vi "Delete TargetPanel by NodeRef.vi"(8 "error in":errorcluster caption="错误输入（无错误）", 9 "Abort VI":bool=TRUE, 10 "Node*":refnum<data-value>, 11 "PanelRootNode 输入":refnum<class "PanelRootNode.lvclass"> caption="DNL_LabVIEW Object in") -> (0 "error out":errorcluster caption="错误输出", 3 "PanelRootNode 输出":refnum<class "PanelRootNode.lvclass"> caption="DNL_LabVIEW Object out")   [LabVIEW 2016, in "PanelRootNode.lvclass"]
uses:
  PanelRootNode.lvclass
  C:/Users/CL/Desktop/ZcDAQprj0811/ZcDAQprj/Modules/DAQ-Display/PanelSplitToolkit/PanelLinkNode/PanelLinkNode.lvclass
  PanelObject/PanelObject.lvclass
  PanelLinkNode/PanelLinkNode.lvclass/PanelLinkNode.ctl
  PanelDataNode/PanelDataNode.lvclass
  C:/Users/CL/Desktop/ZcDAQprj0811/ZcDAQprj/Modules/DAQ-Display/PanelSplitToolkit/PanelObject/PanelObject.lvclass
  PanelLinkNode/PanelLinkNode.lvclass
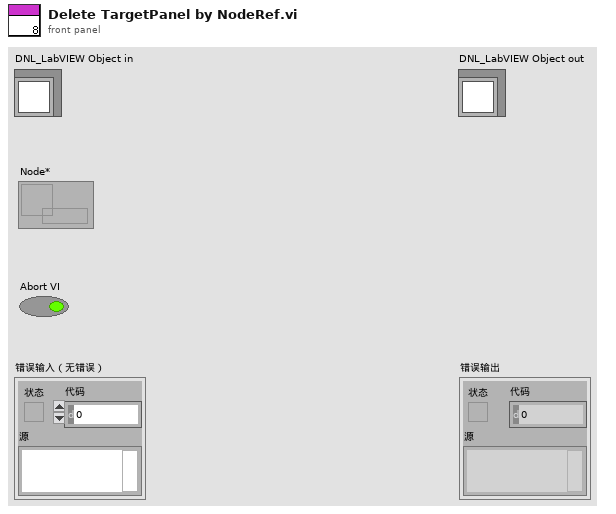
[diagram p1: front panel]
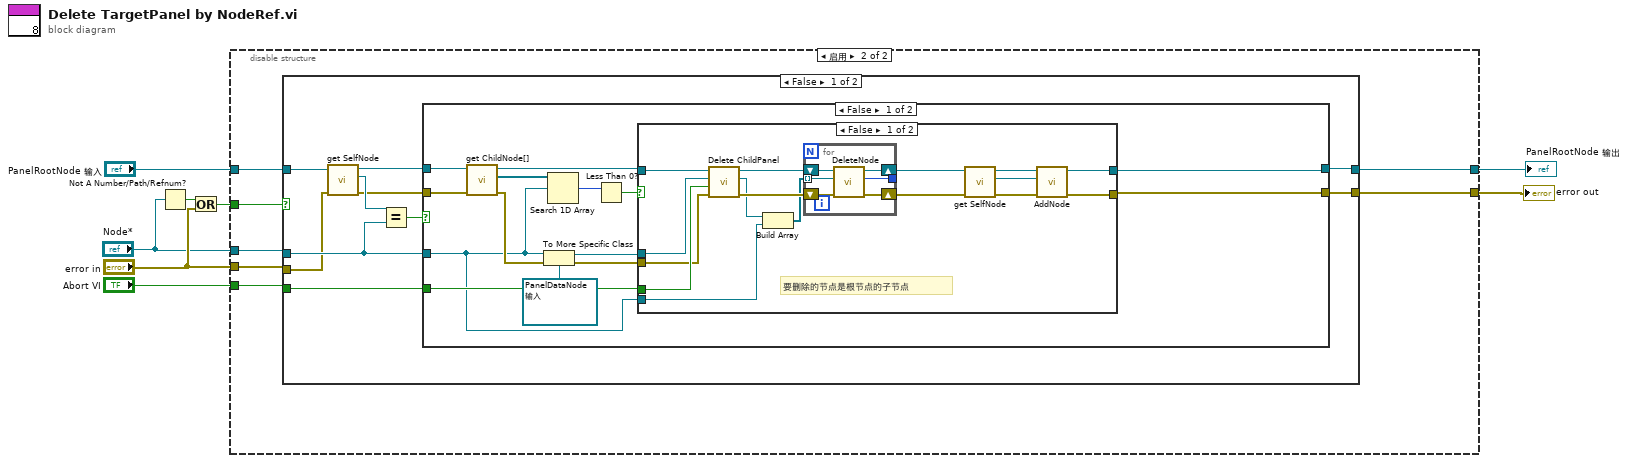
[diagram p0: block diagram]
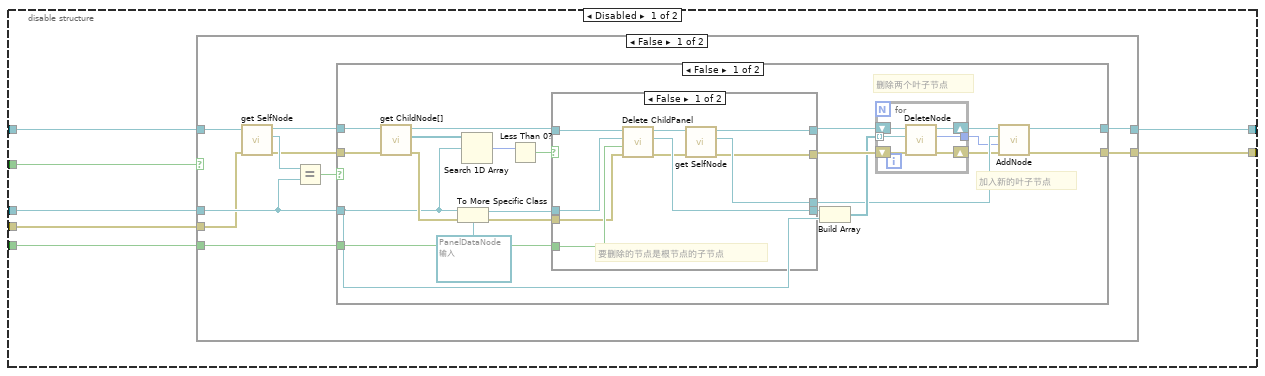
[diagram p2: hidden frame]
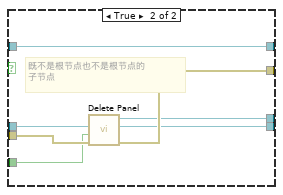
[diagram p3: hidden frame]
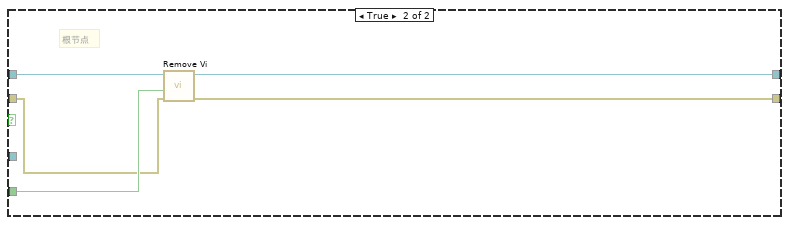
[diagram p4: hidden frame]
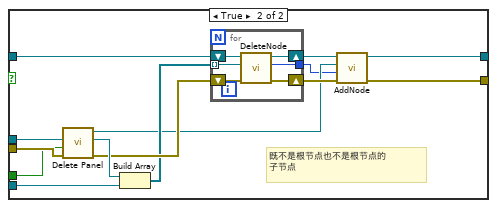
[diagram p6: hidden frame]
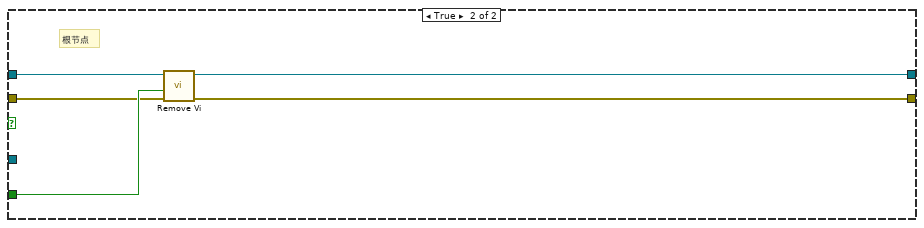
[diagram p7: hidden frame]
diagram:
  n1 = Not A Number/Path/Refnum?(number/path/refnum="Node*") -> (NaN/Path/Refnum?=w5:bool)
  n2 = Or(x=w5, y="error in") -> (x .or. y?=w4:bool)
  n3 = disable-structure shown="启用" {
    disable-tunnel: [w15 w82] -> w8
    disable-tunnel: "PanelRootNode 输入" -> [w14 w84]
    disable-tunnel: [w13 w83] -> w6
    disable-tunnel: w4 -> [w12 w78]
    disable-tunnel: "error in" -> [w11 w81]
    disable-tunnel: "Abort VI" -> [w10 w79]
    disable-tunnel: "Node*" -> [w9 w80]
    frame Disabled {
      n4 = case shown="False" w12 {
        tunnel: [w17 w76] -> w15
        tunnel: [w21 w77] -> w13
        tunnel: w14 -> [w25 w77]
        tunnel: w9 -> [w18 _]
        tunnel: w11 -> [w16 w76]
        tunnel: w10 -> [w20 _]
        frame False {
          n5 = call "get SelfNode.vi"("error in (no error)"=w16, "PanelLinkNode输入"=w25) -> ("error out"=w19:errorcluster, "SelfNode*"=w24:refnum<data-value>, "PanelLinkNode输出"=w23:refnum<class "PanelRootNode.lvclass">)  [unwired: 7 in]
          n6 = Equal?(x=w24, y=w18) -> (x = y?=w22:bool)
          n7 = case shown="False" w22 {
            tunnel: w23 -> [w47 w75]
            tunnel: [w30 w74] -> w21
            tunnel: w20 -> [w41 w73]
            tunnel: w19 -> [w46 w71]
            tunnel: w18 -> [w34 _]
            tunnel: [w26 w72] -> w17
            frame False {
              # "加入新的叶子节点"
              # "删除两个叶子节点"
              n8 = call "get ChildNode[].vi"("error in (no error)"=w46, "PanelLinkNode输入"=w47) -> ("error out"=w38:errorcluster, "ChildNode*[]"=w45:refnum<data-value>[], "PanelLinkNode输出"=w43:refnum<class "PanelRootNode.lvclass">)  [unwired: 7 in]
              n9 = To More Specific Class(target class=refnum<data-value> refnum ("数据值引用"), reference=w34, error in=w38) -> (specific class reference=w39:refnum<data-value>, error out=w37:errorcluster)
              n10 = Search 1D Array(1D array=w45, element=w34) -> (index of element=w44:i32)  [unwired: 1 in]
              n11 = Less Than 0?(x=w44) -> (x < 0?=w42:bool)
              n12 = case shown="False" w42 {
                tunnel: w43 -> [w63 w70]
                tunnel: [w57 w70] -> w36
                tunnel: w39 -> [w62 w69]
                tunnel: w41 -> [w61 w66]
                tunnel: w37 -> [w60 w68]
                tunnel: [w54 w67] -> w33
                tunnel: [w59 w65] -> w35
                tunnel: [w56 w64] -> w29
                frame False {
                  # "要删除的节点是根节点的子节点"
                  n13 = call-dynamic "Delete ChildPanel.vi"("error in"=w60, "Abort VI"=w61, "ChildNode*"=w62, "ParentNode in"=w63) -> ("error out"=w55:errorcluster, "AnotherChildNode*"=w59:refnum<data-value>, "Parent out"=w58:refnum<class "PanelRootNode.lvclass">)  [unwired: 5 in]
                  n14 = call "get SelfNode.vi"("error in (no error)"=w55, "PanelLinkNode输入"=w58) -> ("error out"=w54:errorcluster, "SelfNode*"=w56:refnum<data-value>, "PanelLinkNode输出"=w57:refnum<class "PanelRootNode.lvclass">)  [unwired: 7 in]
                }
                frame True {
                  # "既不是根节点也不是根节点的\n子节点"
                  n15 = call "Delete Panel.vi"("error in"=w68, "Abort VI"=w66, "SelfNode*"=w69) -> ("error out"=w67:errorcluster, "BrotherNodeBeDeleted"=w65:refnum<data-value>, "ParentNode*"=w64:refnum<data-value>)  [unwired: 6 in]
                }
              }
              n16 = Build Array(w35, w34) -> (w32:refnum<data-value>[])
              n17 = for {
                tunnel: w32 -> [w50] mode=indexing
                shift-right: [w52] -> w31
                shift-left: w36 -> [w53]
                shift-right: [w49] -> w27
                shift-left: w33 -> [w51]
                tunnel: [w48] -> w28
                n18 = call "DeleteNode.vi"("error in (no error)"=w51, "Node*"=w50, "PanelRootNode 输入"=w53) -> ("error out"=w49:errorcluster, "index"=w48:i32, "PanelRootNode 输出"=w52:refnum<class "PanelRootNode.lvclass">)  [unwired: 6 in]
              }
              n19 = call "AddNode.vi"("error in (no error)"=w27, "Index"=w28, "Node*"=w29, "PanelRootNode 输入"=w31) -> ("error out"=w26:errorcluster, "PanelRootNode 输出"=w30:refnum<class "PanelRootNode.lvclass">)  [unwired: 6 in]
            }
            frame True {
              # "根节点"
              n20 = call-dynamic "Remove Vi.vi"("error in"=w71, "Abort VI"=w73, "PanelDataNode 输入"=w75) -> ("error out"=w72:errorcluster, "PanelDataNode 输出"=w74:refnum<class "PanelRootNode.lvclass">)  [unwired: 5 in, 2 out]
            }
          }
        }
        frame True {
        }
      }
    }
    frame Enabled {
      n21 = case shown="False" w78 {
        tunnel: [w86 w156] -> w82
        tunnel: [w90 w157] -> w83
        tunnel: w84 -> [w94 w157]
        tunnel: w80 -> [w87 _]
        tunnel: w81 -> [w85 w156]
        tunnel: w79 -> [w89 _]
        frame False {
          n22 = call "get SelfNode.vi"("error in (no error)"=w85, "PanelLinkNode输入"=w94) -> ("error out"=w88:errorcluster, "SelfNode*"=w93:refnum<data-value>, "PanelLinkNode输出"=w92:refnum<class "PanelRootNode.lvclass">)  [unwired: 7 in]
          n23 = Equal?(x=w93, y=w87) -> (x = y?=w91:bool)
          n24 = case shown="False" w91 {
            tunnel: w92 -> [w108 w155]
            tunnel: [w96 w154] -> w90
            tunnel: w89 -> [w102 w153]
            tunnel: w88 -> [w107 w151]
            tunnel: w87 -> [w97 _]
            tunnel: [w95 w152] -> w86
            frame False {
              n25 = call "get ChildNode[].vi"("error in (no error)"=w107, "PanelLinkNode输入"=w108) -> ("error out"=w99:errorcluster, "ChildNode*[]"=w106:refnum<data-value>[], "PanelLinkNode输出"=w104:refnum<class "PanelRootNode.lvclass">)  [unwired: 7 in]
              n26 = To More Specific Class(target class=refnum<data-value> refnum ("数据值引用"), reference=w97, error in=w99) -> (specific class reference=w100:refnum<data-value>, error out=w98:errorcluster)
              n27 = Search 1D Array(1D array=w106, element=w97) -> (index of element=w105:i32)  [unwired: 1 in]
              n28 = Less Than 0?(x=w105) -> (x < 0?=w103:bool)
              n29 = case shown="False" w103 {
                tunnel: w104 -> [w124 w141]
                tunnel: [w109 w133] -> w96
                tunnel: w100 -> [w123 w144]
                tunnel: w102 -> [w122 w142]
                tunnel: w98 -> [w121 w143]
                tunnel: [w110 w134] -> w95
                tunnel: w97 -> [w117 w140]
                frame False {
                  # "要删除的节点是根节点的子节点"
                  n30 = call-dynamic "Delete ChildPanel.vi"("error in"=w121, "Abort VI"=w122, "ChildNode*"=w123, "ParentNode in"=w124) -> ("error out"=w119:errorcluster, "AnotherChildNode*"=w118:refnum<data-value>, "Parent out"=w120:refnum<class "PanelRootNode.lvclass">)  [unwired: 5 in]
                  n31 = Build Array(w118, w117) -> (w116:refnum<data-value>[])
                  n32 = for {
                    tunnel: w116 -> [w127] mode=indexing
                    shift-right: [w129] -> w115
                    shift-left: w120 -> [w130]
                    shift-right: [w126] -> w114
                    shift-left: w119 -> [w128]
                    tunnel: [w125] -> _
                    n33 = call "DeleteNode.vi"("error in (no error)"=w128, "Node*"=w127, "PanelRootNode 输入"=w130) -> ("error out"=w126:errorcluster, "index"=w125:i32, "PanelRootNode 输出"=w129:refnum<class "PanelRootNode.lvclass">)  [unwired: 6 in]
                  }
                  n34 = call "get SelfNode.vi"("error in (no error)"=w114, "PanelLinkNode输入"=w115) -> ("error out"=w111:errorcluster, "SelfNode*"=w112:refnum<data-value>, "PanelLinkNode输出"=w113:refnum<class "PanelRootNode.lvclass">)  [unwired: 7 in]
                  n35 = call "AddNode.vi"("error in (no error)"=w111, "Node*"=w112, "PanelRootNode 输入"=w113) -> ("error out"=w110:errorcluster, "PanelRootNode 输出"=w109:refnum<class "PanelRootNode.lvclass">)  [unwired: 7 in]
                }
                frame True {
                  # "既不是根节点也不是根节点的\n子节点"
                  n36 = call "Delete Panel.vi"("error in"=w143, "Abort VI"=w142, "SelfNode*"=w144) -> ("error out"=w138:errorcluster, "BrotherNodeBeDeleted"=w139:refnum<data-value>, "ParentNode*"=w132:refnum<data-value>)  [unwired: 6 in]
                  n37 = Build Array(w139, w140) -> (w137:refnum<data-value>[])
                  n38 = for {
                    tunnel: w137 -> [w147] mode=indexing
                    shift-right: [w149] -> w136
                    shift-left: w141 -> [w150]
                    shift-right: [w146] -> w135
                    shift-left: w138 -> [w148]
                    tunnel: [w145] -> w131
                    n39 = call "DeleteNode.vi"("error in (no error)"=w148, "Node*"=w147, "PanelRootNode 输入"=w150) -> ("error out"=w146:errorcluster, "index"=w145:i32, "PanelRootNode 输出"=w149:refnum<class "PanelRootNode.lvclass">)  [unwired: 6 in]
                  }
                  n40 = call "AddNode.vi"("error in (no error)"=w135, "Index"=w131, "Node*"=w132, "PanelRootNode 输入"=w136) -> ("error out"=w134:errorcluster, "PanelRootNode 输出"=w133:refnum<class "PanelRootNode.lvclass">)  [unwired: 6 in]
                }
              }
            }
            frame True {
              # "根节点"
              n41 = call-dynamic "Remove Vi.vi"("error in"=w151, "Abort VI"=w153, "PanelDataNode 输入"=w155) -> ("error out"=w152:errorcluster, "PanelDataNode 输出"=w154:refnum<class "PanelRootNode.lvclass">)  [unwired: 5 in, 2 out]
            }
          }
        }
        frame True {
        }
      }
    }
  }
  "error out" <- w8
  "PanelRootNode 输出" <- w6
